vi "Assign-Serial-Number-sql.vi"(9 "CSV path":path=path "C:/LNK213-300/Serial_Log.csv", 10 "Test Operator ID":string="13984", 11 "PCBA Barcode":string="SVI77664916000003") -> (0 "Table":string[][](table), 1 "Record Found":bool, 2 "Serial Number (STR)":string, 3 "Serial Number (NUM)":i32)   [LabVIEW 2011]
uses:
  <vilib>/Utility/file.llb/Write To Spreadsheet File (string).vi
panel:
  out "Table 2":string[][](table)
  out "String 3":string
  out "String 2":string
  out "unsigned 16bit integer":u16[](array[numeric])
  out "Summing of first four bytes BIN":i8 format="%b"
  out "hex integer string":string
  out "Loop":i32
  out "result string":string
  out "crc":string
  out "8digi":string
  out "Data":string[][](array[string])
  in  "Error in (no error)":errorcluster
  out "Error out":errorcluster
  out "Found  SN in Index":i32[](array[numeric])
  out "Last Serial Number":i32
  out "Last Record":i32
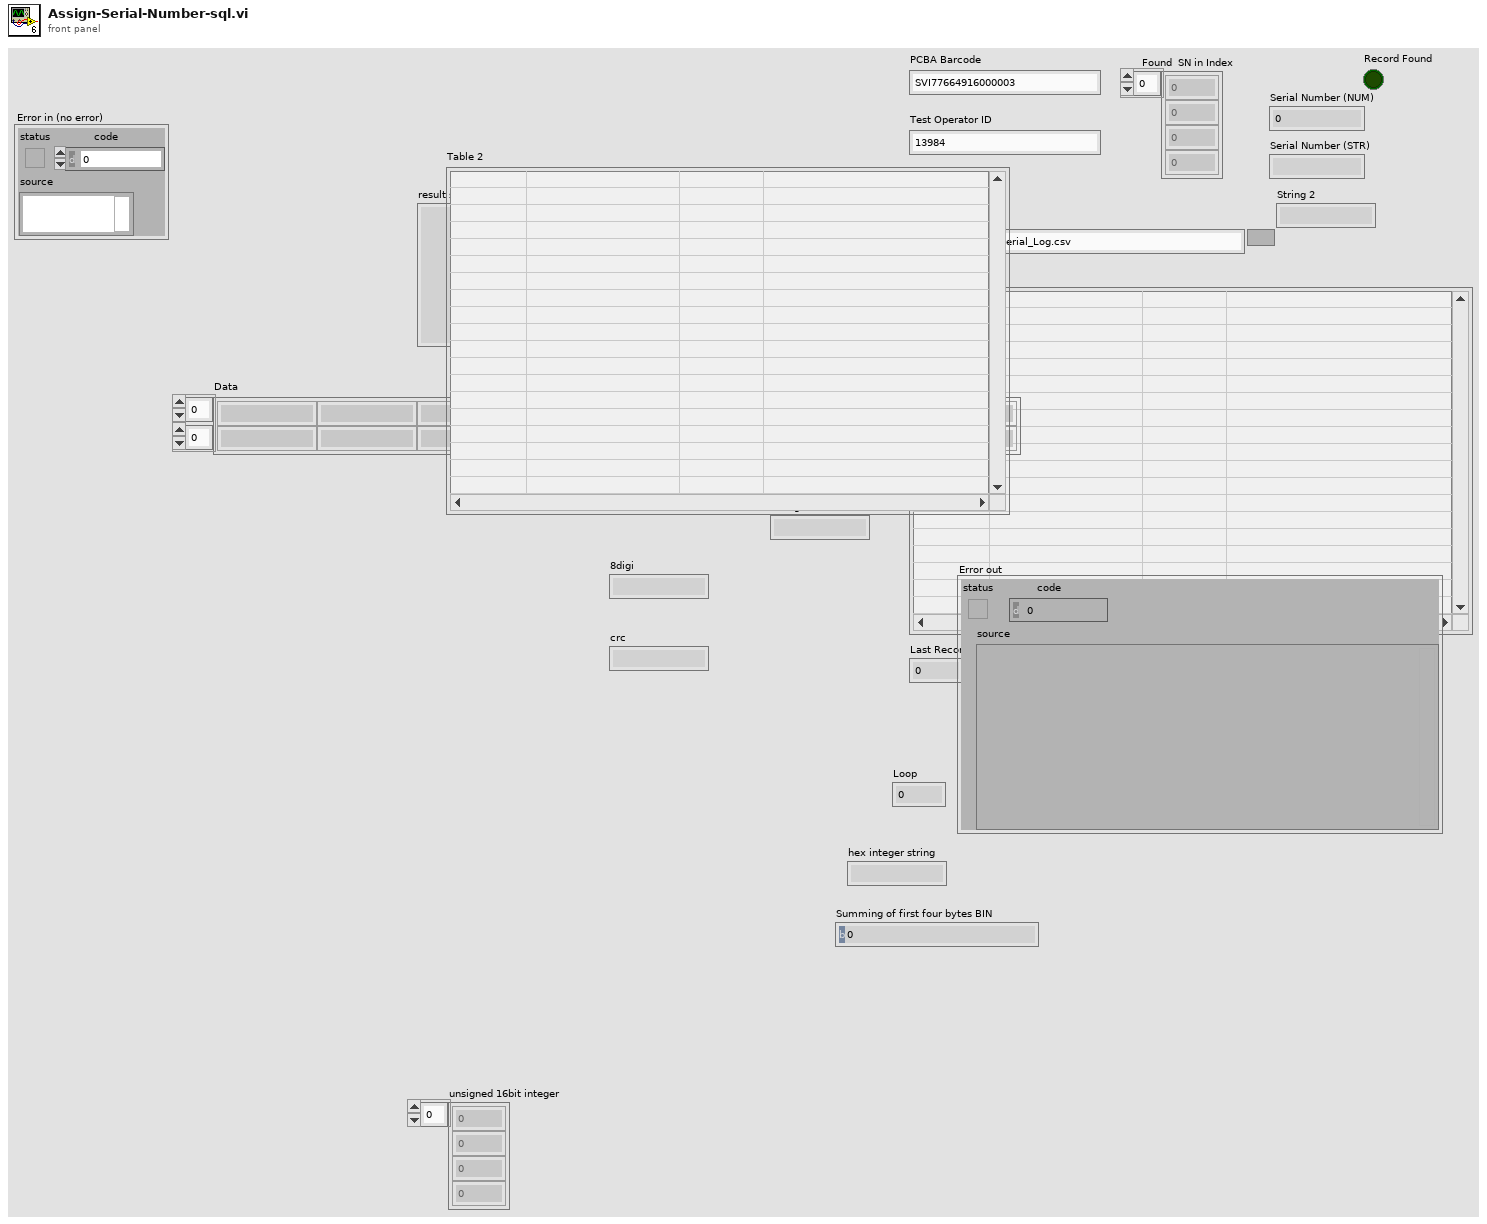
[diagram p1: front panel]
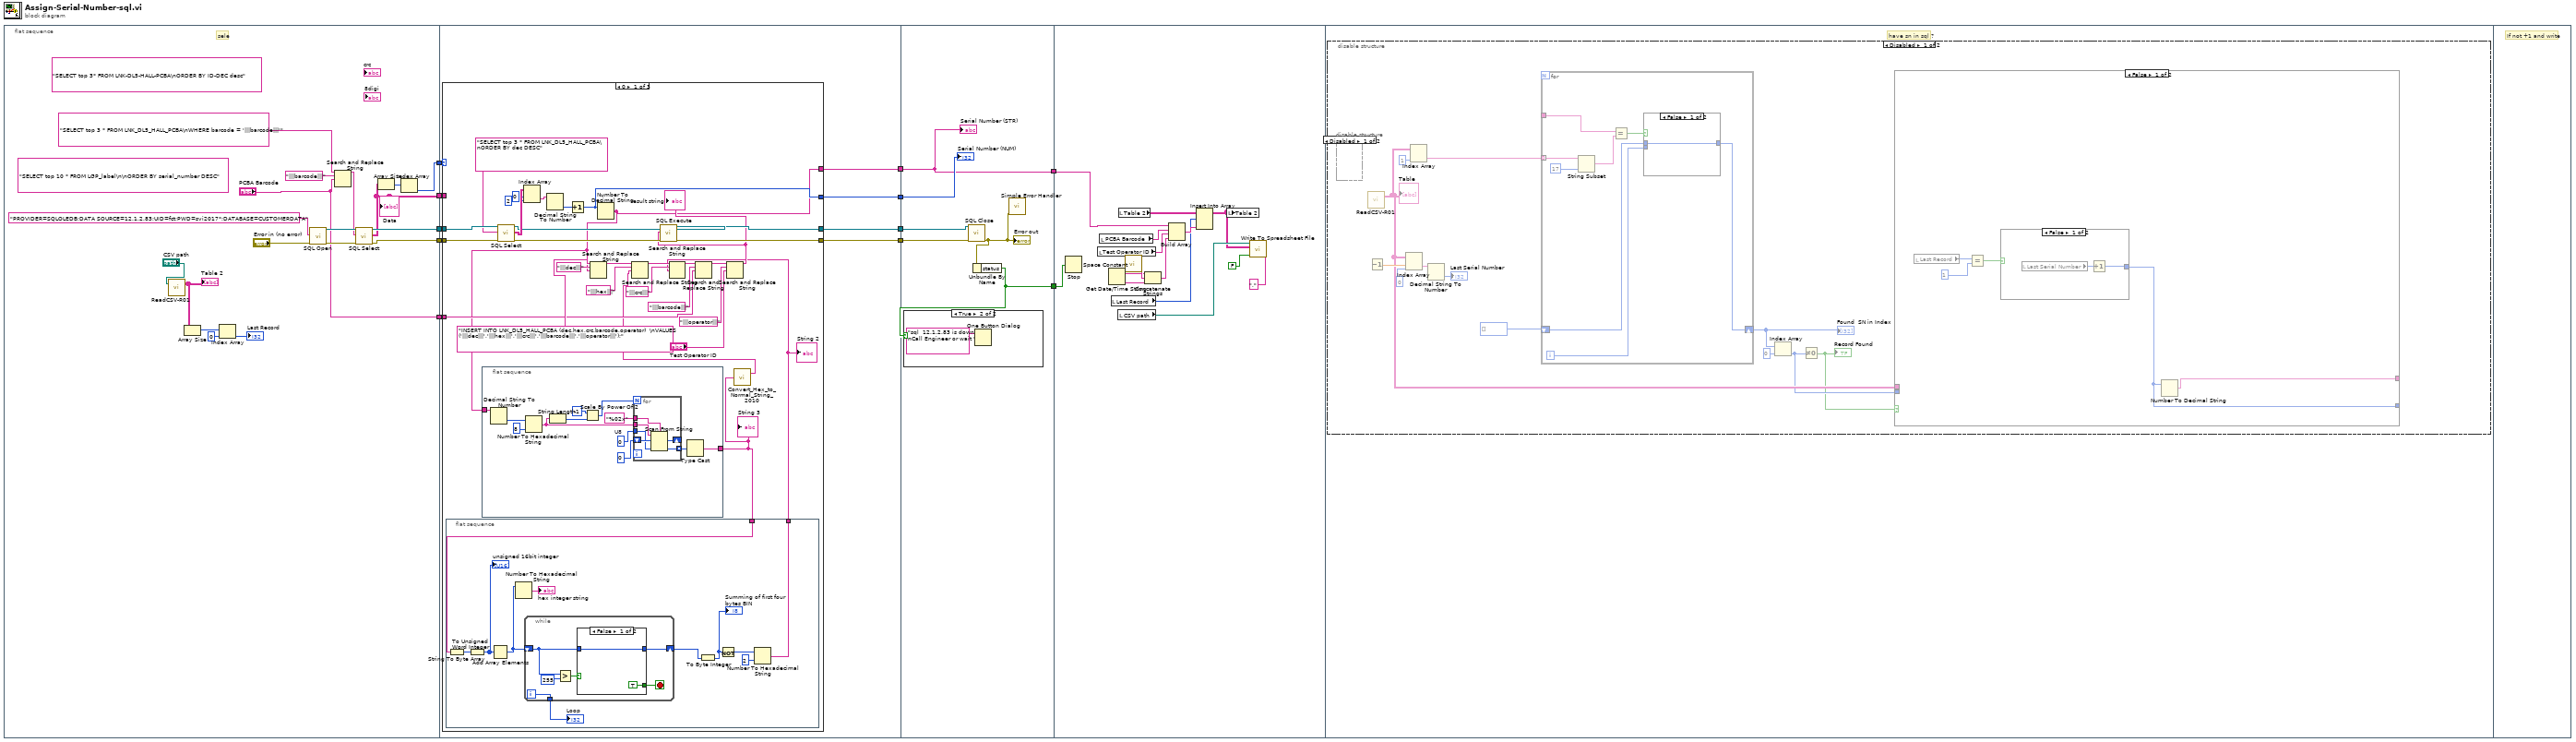
[diagram p0: block diagram]
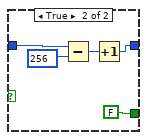
[diagram p2: hidden frame]
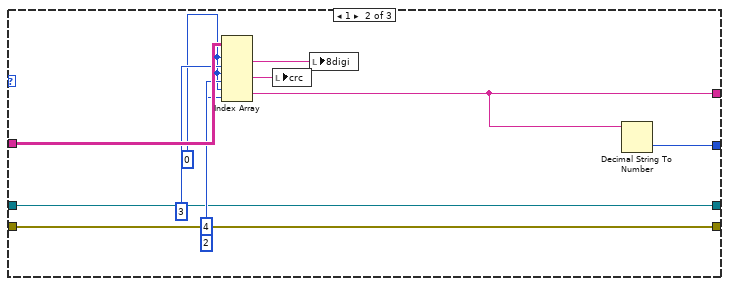
[diagram p3: hidden frame]
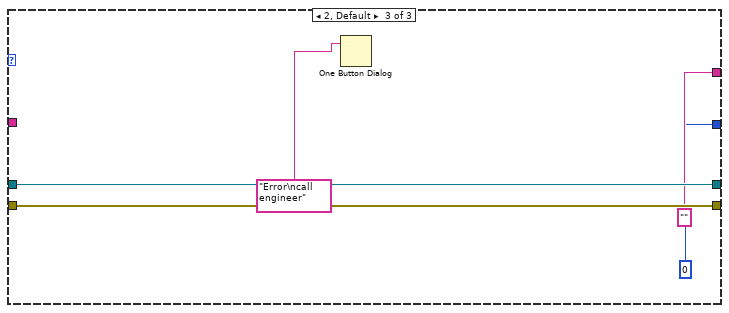
[diagram p4: hidden frame]
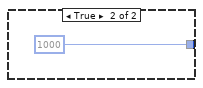
[diagram p7: hidden frame]
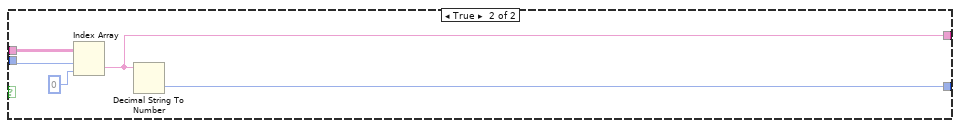
[diagram p8: hidden frame]
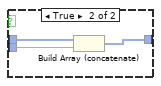
[diagram p9: hidden frame]
diagram:
  n1 = flat-sequence {
    tunnel: [w22] -> w11
    tunnel: [w21] -> w9
    tunnel: [w19] -> w7
    tunnel: [w18] -> w6
    tunnel: ["PCBA Barcode"] -> w5
    tunnel: w11 -> [w33]
    tunnel: [w34] -> w10
    tunnel: w9 -> [w36]
    tunnel: [w35] -> w8
    tunnel: w7 -> [w38]
    tunnel: w6 -> [w37]
    tunnel: w5 -> [w32]
    tunnel: [w31] -> w4
    tunnel: [w30] -> w3
    tunnel: w10 -> [w132]
    tunnel: w8 -> [w131]
    tunnel: w4 -> [w129]
    tunnel: w3 -> [w130]
    tunnel: [w129] -> w2
    tunnel: [w127] -> w1
    tunnel: w2 -> [w135]
    tunnel: w1 -> [w134]
    frame #0 {
      (unwired) "SELECT top 3* FROM LNK-DL5-HALL-PCBA\nORDER BY ID-DEC desc" ("SQL Query 2")
      (unwired) "SELECT top 10 * FROM LGP_label\n\nORDER BY serial_number DESC" ("SQL Query 2")
      # "sele"
      n2 = call "ReadCSV-R01.vi"("CSV path"="CSV path") -> ("Table"=w12:string[][])  [unwired: 1 in, 1 out]
      "Table 2" <- w12
      n3 = Array Size(array=w12) -> (size(s)=w13:i32[])
      n4 = Index Array(array=w13, index=0) -> (element=→"Last Record":i32)
      n5 = call "SQL Open.vi"("ConnectionString In"="PROVIDER=SQLOLEDB;DATA SOURCE=12.1.2.83;UID=fct;PWD=svi2017*;DATABASE=CUSTOMERDATA" ("regular expression"), "Error in (no error)"="Error in (no error)") -> ("Connection Out"=w29:refnum<k7>, "Error out"=w28:errorcluster)  [unwired: 16 in]
      n6 = Search and Replace String(input string="SELECT top 3 * FROM LNK_DL5_HALL_PCBA\nWHERE barcode = '|||barcode|||'" ("SQL Query 2"), search string="|||barcode|||", replace string="PCBA Barcode") -> (result string=w25:string)  [unwired: 5 in, 3 out]
      n7 = call "SQL Select.vi"("Connection In"=w29, "SQL Query"=w25, "Error in (no error)"=w28) -> ("Connection Out"=w22:refnum<k7>, "Data"=w18:string[][], "Error out"=w21:errorcluster)  [unwired: 14 in]
      "Data" <- w18
      n8 = Array Size(array=w18) -> (size(s)=w20:i32[])
      n9 = Index Array(array=w20) -> (element=w19:i32)  [unwired: 1 in]
    }
    frame #1 {
      n10 = case shown="0" w38 {
        tunnel: w37 -> [_ w121 _]
        tunnel: w36 -> [w67 w116 w126]
        tunnel: [w57 w116 w126] -> w35
        tunnel: [w59 w115 w125] -> w34
        tunnel: w33 -> [w68 w115 w125]
        tunnel: w32 -> [w46 _ _]
        tunnel: [w42 w112 "" ("String")] -> w31
        tunnel: [w43 w111 0] -> w30
        frame 0 {
          n11 = flat-sequence {
            tunnel: w40 -> [w71]
            tunnel: [w70] -> w41
            frame #0 {
              n12 = String To Byte Array(string=w71) -> (unsigned byte array=w72:u8[])
              n13 = To Unsigned Word Integer(number=w72) -> (unsigned 16bit integer=w73:u16[])
              "unsigned 16bit integer" <- w73
              n14 = Add Array Elements(numeric array=w73) -> (sum=w77:u16)
              n15 = Number To Hexadecimal String(2:w77) -> (0:→"hex integer string":string)  [unwired: 1 in]
              n16 = while {
                shift-right: [w83] -> w78
                shift-left: w77 -> [w82]
                tunnel: [w80] -> w79
                i -> [w80]
                stop <- w81 stop-if-true
                n17 = Greater?(x=w82, y=u16 255) -> (0:w85:bool)
                n18 = case shown="False" w85 {
                  tunnel: [w87 w88] -> w83
                  tunnel: w82 -> [w87 w91]
                  tunnel: [TRUE FALSE] -> w81
                  frame False {
                  }
                  frame True {
                    n19 = Subtract(x=w91, y=u16 256) -> (x-y=w89:u16)
                    n20 = Increment(x=w89) -> (x+1=w88:u16)
                  }
                }
              }
              "Loop" <- w79
              n21 = To Byte Integer(number=w78) -> (8bit integer=w76:i8)
              "Summing of first four bytes BIN" <- w76
              n22 = Not(x=w76) -> (.not. x?=w75:i8)
              n23 = Number To Hexadecimal String(1:i16 2 ("width (-)"), 2:w75) -> (0:w70:string)
            }
          }
          n24 = flat-sequence {
            tunnel: w42 -> [w94]
            tunnel: [w93] -> w40
            frame #0 {
              w98 = u8 0  # U8
              n25 = Decimal String To Number(string=w94) -> (number=w95:i32)  [unwired: 2 in, 1 out]
              n26 = Number To Hexadecimal String(1:i16 8 ("width (-)"), 2:w95) -> (0:w104:string)
              n27 = String Length(string=w104) -> (length=w101:i32)
              n28 = Scale By Power Of 2(n=-1, x=w101) -> (x*2^n=w103:i32)
              n29 = for {
                N: w103 -> [_]
                shift-right: [w109] -> _
                shift-left: u32 0 -> [w110]
                tunnel: w104 -> [w108]
                tunnel: w98 -> [w107]
                tunnel: [w106] -> w99 mode=indexing
                tunnel: "%02x" ("format string") -> [w105]
                n30 = Scan From String(format string=w105, input string=w108, initial scan location=w110, default 1=w107) -> (offset past scan=w109:u32, output 1=w106:u8)  [unwired: 1 in, 2 out]
              }
              n31 = Type Cast(x=w99) -> (*(type *) &x=w93:string)  [unwired: 1 in]
            }
          }
          n32 = call "SQL Select.vi"("Connection In"=w68, "SQL Query"="SELECT top 3 * FROM LNK_DL5_HALL_PCBA\nORDER BY dec DESC" ("SQL Query 2"), "Error in (no error)"=w67) -> ("Connection Out"=w60:refnum<k7>, "Data"=w65:string[][], "Error out"=w58:errorcluster)  [unwired: 14 in]
          n33 = Index Array(array=w65, index (row)=0, index (col)=2 ("disabled index (col)")) -> (element=w62:string)
          n34 = Decimal String To Number(string=w62) -> (number=w61:i32)  [unwired: 2 in, 1 out]
          n35 = Increment(x=w61) -> (x+1=w43:i32)
          n36 = Number To Decimal String(number=w43) -> (decimal integer string=w42:string)  [unwired: 1 in]
          n37 = Search and Replace String(input string="INSERT INTO LNK_DL5_HALL_PCBA (dec,hex,crc,barcode,operator)  \nVALUES ('|||dec|||','|||hex|||','|||crc|||','|||barcode|||','|||operator|||');" ("replace string (\"\")"), search string="|||dec|||", replace string=w42) -> (result string=w55:string)  [unwired: 5 in, 3 out]
          n38 = call "Convert_Hex_to_Normal_String_2010.vi"("Initial Hex String"=w40) -> ("Normal String - Number to Hexadecimal String Method"=w39:string)  [unwired: 1 out]
          n39 = Search and Replace String(input string=w55, search string="|||hex|||", replace string=w39) -> (result string=w54:string)  [unwired: 5 in, 3 out]
          n40 = Search and Replace String(input string=w54, search string="|||crc|||", replace string=w41) -> (result string=w53:string)  [unwired: 5 in, 3 out]
          n41 = Search and Replace String(input string=w53, search string="|||barcode|||", replace string=w46) -> (result string=w52:string)  [unwired: 5 in, 3 out]
          n42 = Search and Replace String(input string=w52, search string="|||operator|||", replace string="Test Operator ID") -> (result string=w51:string)  [unwired: 5 in, 3 out]
          "result string" <- w51
          n43 = call "SQL Execute.vi"("Connection In"=w60, "SQL Query"=w51, "Error in (no error)"=w58) -> ("Connection Out"=w59:refnum<k7>, "Error out"=w57:errorcluster)  [unwired: 15 in]
          "String 2" <- w41
          "String 3" <- w40
        }
        frame 1 {
          w114 = 0 ("index (row)")
          n44 = Index Array(array=w121, index (row) #1=w114, index (col) #1=3 ("disabled index (col)"), index (row) #2=w114, index (col) #2=4 ("disabled index (col)"), index (row) #3=w114, index (col) #3=2 ("disabled index (col)")) -> (element #1=w117:string, element #2=w118:string, element #3=w112:string)
          n45 = local write "crc"(w118) -> ()
          n46 = local write "8digi"(w117) -> ()
          n47 = Decimal String To Number(string=w112) -> (number=w111:i32)  [unwired: 2 in, 1 out]
        }
        frame 2, Default {
          n48 = One Button Dialog(message="Error\ncall engineer") -> ()  [unwired: 1 in, 1 out]
        }
      }
    }
    frame #2 {
      n49 = call "SQL Close.vi"("Connection In"=w132, "Error in (no error)"=w131) -> ("Error out"=w128:errorcluster)  [unwired: 17 in]
      "Error out" <- w128
      n50 = Unbundle By Name(w128) -> ("status"=w127:bool)
      n51 = case shown="True" w127 {
        frame False {
        }
        frame True {
          n52 = One Button Dialog(message="sql  12.1.2.83 is down\nCall Engineer or wait ") -> ()  [unwired: 1 in, 1 out]
        }
      }
      n53 = call <vilib>:"Simple Error Handler.vi"("error in (no error)"=w128) -> ()  [unwired: 4 in, 5 out]
      "Serial Number (NUM)" <- w130
      "Serial Number (STR)" <- w129
    }
    frame #3 {
      n54 = Stop(stop? (T)=w134) -> ()
      n55 = local read "Test Operator ID"() -> (w144:string)
      n56 = local read "PCBA Barcode"() -> (w140:string)
      n57 = Get Date/Time String() -> (date string=w145:string, time string=w146:string)  [unwired: 3 in]
      n58 = local read "Last Record"() -> (w138:i32)
      n59 = local read "CSV path"() -> (w143:path)
      n60 = local read "Table 2"() -> (w137:string[][])
      n61 = call <vilib>:"Space Constant.vi"() -> ("String"=w147:string)
      n62 = Concatenate Strings(w145, w147, w146) -> (w148:string)
      n63 = Build Array(w135, w140, w144, w148) -> (w139:string[])
      n64 = Insert Into Array(array=w137, index (row)=w138, new element=w139) -> (w141:string[][])  [unwired: 1 in]
      n65 = local write "Table 2"(w141) -> ()
      n66 = call-poly <vilib>:"Write To Spreadsheet File.vi"("delimiter (\\t)"="," ("delimiter (\\t)"), "append to file? (new file:F)"=FALSE, "2D data"=w141, "file path (dialog if empty)"=w143) -> ()  [unwired: 4 in, 1 out]
    }
    frame #4 {
      # "have sn in sql ?"
      n67 = disable-structure shown="Disabled" {
        frame Disabled {
          n68 = disable-structure shown="Disabled" {
            frame Disabled {
            }
            frame Enabled {
            }
          }
          n69 = call "ReadCSV-R01.vi"() -> ("Table"=w154:string[][], "CSV path"=w149:path)  [unwired: 1 in, 1 out]
          "Table" <- w154
          n70 = Decrement() -> (x=w160:dbl, x-1=w161:dbl)
          n71 = Index Array(array=w154, index (row)=w161, index (col)=0 ("disabled index (col)")) -> (element=w159:string)
          n72 = Index Array(array=w154, index (col)=1 ("disabled index (col)")) -> (element=w157:string[])  [unwired: 1 in]
          n73 = Decimal String To Number(string=w159) -> (number=→"Last Serial Number":i32)  [unwired: 2 in, 1 out]
          n74 = for {
            tunnel: _ -> [w180]
            tunnel: w157 -> [w183] mode=indexing
            shift-right: [w176] -> w153
            shift-left: i32[] [] -> [w178]
            i -> [w177]
            n75 = String Subset(string=w183, length (rest)=17 ("disabled index (col)")) -> (substring=w181:string)  [unwired: 1 in]
            n76 = Equal?(x=w180, y=w181) -> (x = y?=w179:bool)
            n77 = case shown="False" w179 {
              tunnel: [w184 w187] -> w176
              tunnel: w178 -> [w184 w186]
              tunnel: w177 -> [_ w185]
              frame False {
              }
              frame True {
                n78 = Build Array (concatenate)(w186, w185) -> (w187:i32[])
              }
            }
          }
          "Found  SN in Index" <- w153
          n79 = Index Array(array=w153, index=0) -> (element=w151:i32)
          n80 = Not Equal To 0?(x=w151) -> (x != 0?=w150:bool)
          "Record Found" <- w150
          n81 = case shown="False" w150 {
            tunnel: w154 -> [_ w175]
            tunnel: w151 -> [_ w173]
            tunnel: [w163 w172] -> _
            tunnel: [w167 w171] -> _
            frame False {
              n82 = local read "Last Record"() -> (w166:i32)
              n83 = Equal?(x=w166, y=1 ("index")) -> (x = y?=w164:bool)
              n84 = case shown="False" w164 {
                tunnel: [w168 1000 ("index")] -> w163
                frame False {
                  n85 = local read "Last Serial Number"() -> (w169:i32)
                  n86 = Increment(x=w169) -> (x+1=w168:i32)
                }
                frame True {
                }
              }
              n87 = Number To Decimal String(number=w163) -> (decimal integer string=w167:string)  [unwired: 1 in]
            }
            frame True {
              n88 = Index Array(array=w175, index (row)=w173, index (col)=0 ("disabled index (row)")) -> (element=w171:string)
              n89 = Decimal String To Number(string=w171) -> (number=w172:i32)  [unwired: 2 in, 1 out]
            }
          }
        }
        frame Enabled {
        }
      }
    }
    frame #5 {
      # "If not +1 and write"
    }
  }
